vi "Configure Standard Waveform.vi"(0 "VISA resource name":refnum<visa-resource-name>, 1 "Frequency (1000 Hz)":dbl=1000.0, 5 "Channel (0: Channel 1)":u16(ring) items=["Channel 1", "Channel 2"], 7 "Waveform Function (0: Sine)":u16(ring) items=["Sine", "Square", "Pulse", "Ramp", "Noise", "DC", "Sin(x)/x", "Gaussian", "Lorentz", "Exponential Rise", "Exponential Decay", "Haversine"], 9 "Amplitude (1 Vpp)":dbl=1.0, 11 "error in (no error)":errorcluster, 12 "DC Offset (0.00 V)":dbl, 13 "Phase Level (-1)":dbl=-1.0, 14 "Phase Unit (0: Radian)":u16(ring) items=["Radians", "Degrees"]) -> (4 "VISA resource name out":refnum<visa-resource-name>, 15 "error out":errorcluster)   [LabVIEW 2018, in "AWG.lvlib" / "Tektronix AFG 3000 Series.lvlib"]
doc: "Selects the waveform shape, frequency, amplitude, offset, and phase for a standard waveform."
uses:
  Tektronix AFG 3000 Series.lvlib
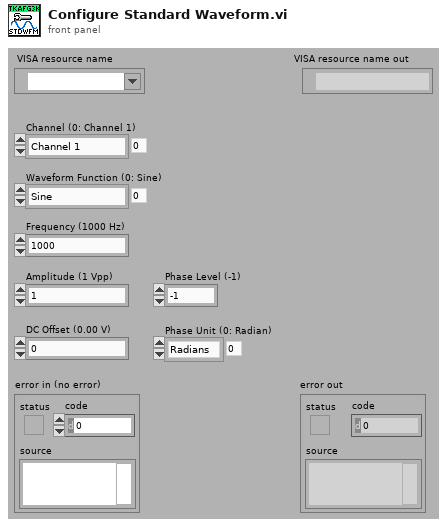
[diagram p1: front panel]
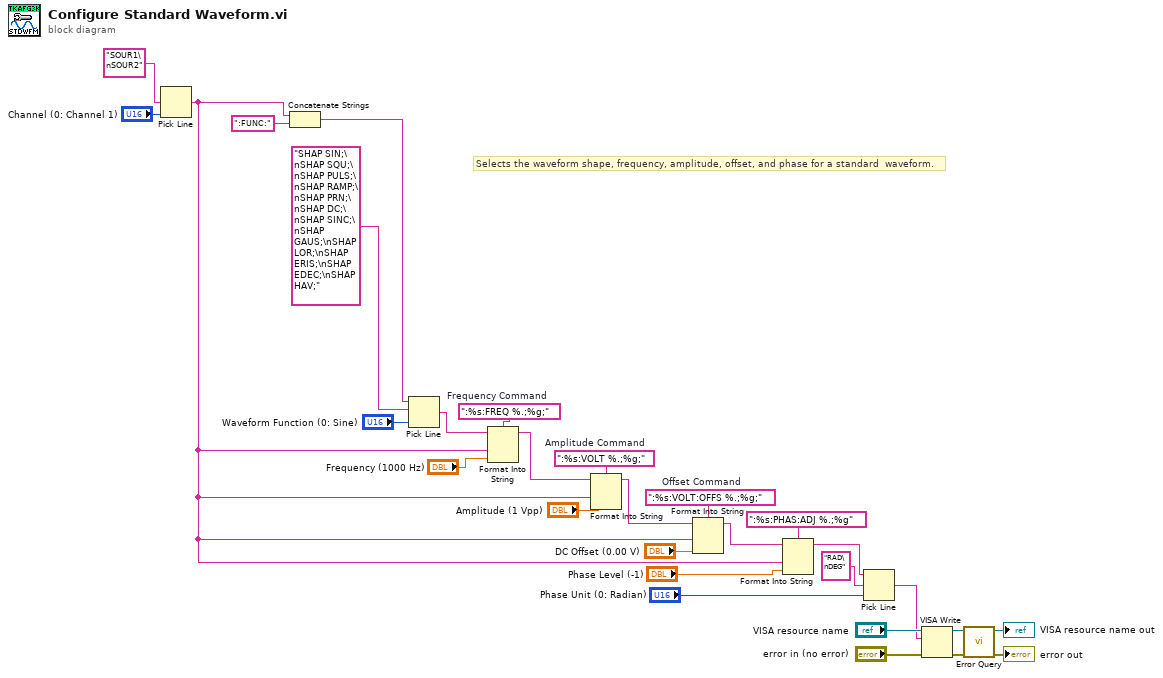
[diagram p0: block diagram]
diagram:
  w18 = ":%s:VOLT:OFFS %.;%g;"  # Offset Command
  w19 = ":%s:VOLT %.;%g;"  # Amplitude Command
  w21 = ":%s:FREQ %.;%g;"  # Frequency Command
  # "Selects the waveform shape, frequency, amplitude, offset, and phase for a standard  waveform."
  n1 = Pick Line(multi-line string="SOUR1\nSOUR2" ("string (\"\")"), line index="Channel (0: Channel 1)") -> (output string=w4:string)  [unwired: 1 in]
  n2 = Concatenate Strings(w4, ":FUNC:" ("string")) -> (w12:string)
  n3 = Pick Line(string ("")=w12, multi-line string="SHAP SIN;\nSHAP SQU;\nSHAP PULS;\nSHAP RAMP;\nSHAP PRN;\nSHAP DC;\nSHAP SINC;\nSHAP GAUS;\nSHAP LOR;\nSHAP ERIS;\nSHAP EDEC;\nSHAP HAV;" ("Function Command"), line index="Waveform Function (0: Sine)") -> (output string=w20:string)
  n4 = Format Into String(format string=w21, initial string=w20, w4, "Frequency (1000 Hz)") -> (resulting string=w16:string)  [unwired: 1 in, 1 out]
  n5 = Format Into String(format string=w19, initial string=w16, w4, "Amplitude (1 Vpp)") -> (resulting string=w17:string)  [unwired: 1 in, 1 out]
  n6 = Format Into String(format string=w18, initial string=w17, w4, "DC Offset (0.00 V)") -> (resulting string=w5:string)  [unwired: 1 in, 1 out]
  n7 = Format Into String(format string=":%s:PHAS:ADJ %.;%g", initial string=w5, w4, "Phase Level (-1)") -> (resulting string=w6:string)  [unwired: 1 in, 1 out]
  n8 = Pick Line(string ("")=w6, multi-line string="RAD\nDEG", line index="Phase Unit (0: Radian)") -> (output string=w1:string)
  n9 = VISA Write(VISA resource name="VISA resource name", write buffer=w1, error in (no error)="error in (no error)") -> (VISA resource name out=w25:refnum<visa-resource-name>, error out=w24:errorcluster)  [unwired: 1 out]
  n10 = call "Error Query.vi"("error in (no error)"=w24, "VISA resource name"=w25) -> ("error out"=→"error out":errorcluster, "VISA resource name out"=→"VISA resource name out":refnum<visa-resource-name>)  [unwired: 6 in, 2 out]
